vi "Read Number of ROIs and Type.vi"(11 "Experimental Folder":path) -> (1 "Patches in Experiment":i32, 2 "Predominant ROI type":T2=enum."Comp. volume", 3 "Imaging Protocol":T1)   [LabVIEW 2017]
uses:
  Typedefs/ROI ID Enum.ctl
  Typedefs/Imaging Protocols enum.ctl
  <vilib>/Utility/file.llb/Read From Spreadsheet File (I64).vi
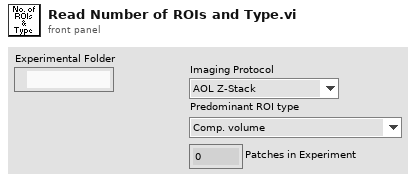
[diagram p1: front panel]
types:
  T1 = typedef "Imaging Protocols enum.ctl" = enum16{"AOL Z-Stack", "Motor Z Stack", "Functional Acquisition", "Single Plane Acquisition", "Volume Acquisition", "Live Imaging", "Live Plane Imaging", "Live Volume Imaging"}
  T2 = typedef "ROI ID Enum.ctl" = enum16{"Point", "MiniScan", "Comp. MiniScan", "Rectangle", "Comp. volume", "Arb. plane point"}
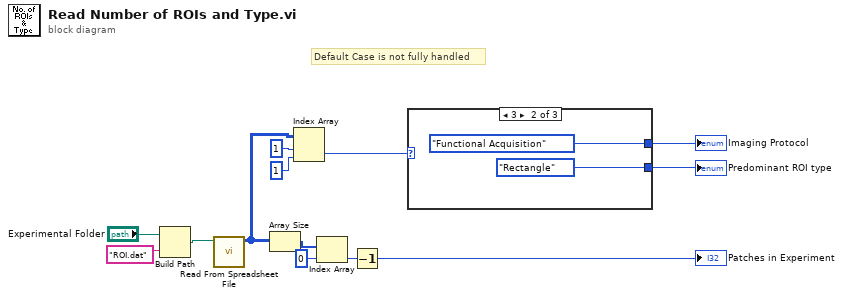
[diagram p0: block diagram]
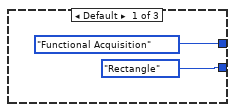
[diagram p2: hidden frame]
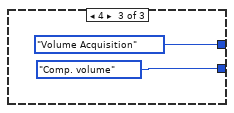
[diagram p3: hidden frame]
diagram:
  # "Default Case is not fully handled"
  n1 = Build Path(base path="Experimental Folder", name or relative path="ROI.dat") -> (appended path=w9:path)
  n2 = call-poly <vilib>:"Read From Spreadsheet File.vi"("file path (dialog if empty)"=w9) -> ("all rows"=w11:i64[][])  [unwired: 6 in, 4 out]
  n3 = Array Size(array=w11) -> (size(s)=w8:i32[])
  n4 = Index Array(array=w11, index (row)=1 ("disabled index (row)"), index (col)=1 ("disabled index (col)")) -> (element=w12:i64)
  n5 = Index Array(array=w8, index=0) -> (element=w6:i32)
  n6 = Decrement(x=w6) -> (x-1=→"Patches in Experiment":i32)
  n7 = case shown="3" w12 {
    tunnel: [Imaging_Protocols_enum."Functional Acquisition" ("Imaging Protocol") Imaging_Protocols_enum."Functional Acquisition" ("Imaging Protocol") Imaging_Protocols_enum."Volume Acquisition" ("Imaging Protocol")] -> w1
    tunnel: [ROI_ID_Enum."Rectangle" ("Predominant ROI type") ROI_ID_Enum."Rectangle" ("Predominant ROI type") ROI_ID_Enum."Comp. volume" ("Predominant ROI type")] -> w2
    frame Default {
    }
    frame 3 {
    }
    frame 4 {
    }
  }
  "Predominant ROI type" <- w2
  "Imaging Protocol" <- w1
